vi "Create_Iteration_Data_Files.vi"(7 "Current Iteration":u32, 8 "error in (no error)":errorcluster, 9 "Counter (in)":refnum<class "Counter.lvclass">, 10 "Hamamatsu_C9100-13 (in)":refnum<class "Hamamatsu_C9100-13.lvclass">, 11 "ExperimentVariables in":refnum<class "ExperimentVariables.lvclass">) -> (0 "error out":errorcluster, 1 "Counter out":refnum<class "Counter.lvclass">, 2 "Hamamatsu_C9100-13":refnum<class "Hamamatsu_C9100-13.lvclass">, 3 "ExperimentVariables out":refnum<class "ExperimentVariables.lvclass">)   [LabVIEW 2013]
uses:
  Camera/Hamamatsu_C9100-13/Hamamatsu_C9100-13.lvclass
  Counter/Counter.lvclass
  ExperimentVariables.lvclass
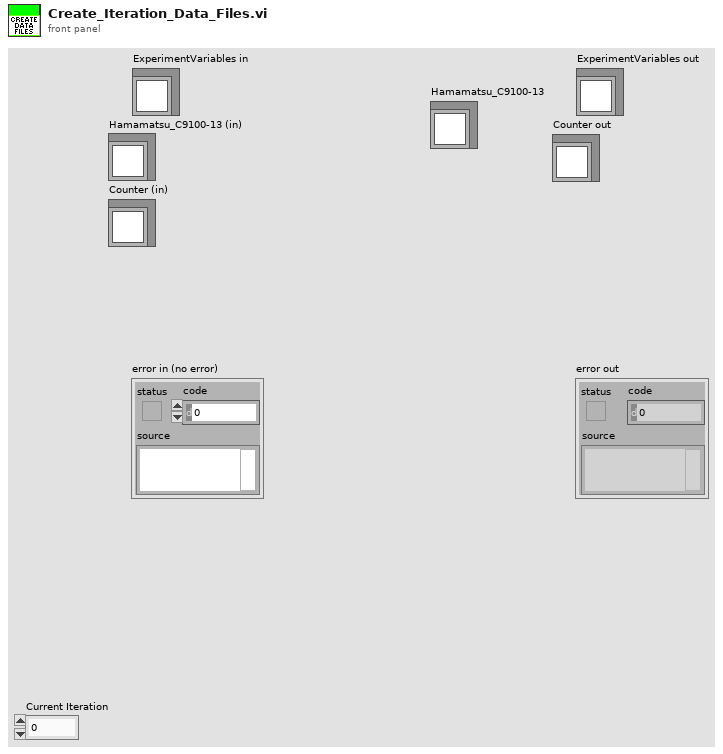
[diagram p1: front panel]
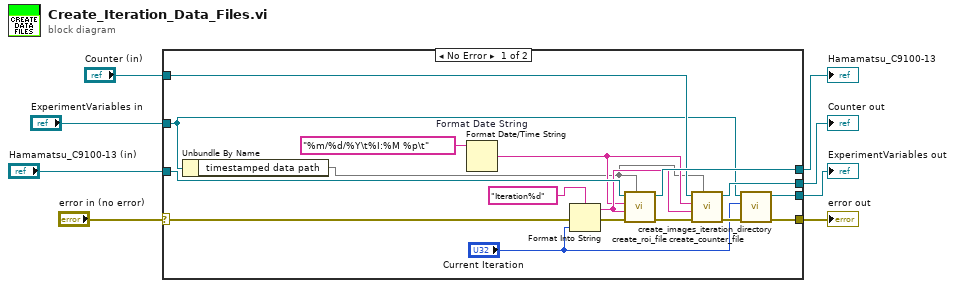
[diagram p0: block diagram]
diagram:
  n1 = case shown="No Error" "error in (no error)" {
    selector: "error in (no error)" -> [w9 w29]
    tunnel: [w14 w29] -> w7
    tunnel: [w12 w28] -> w5
    tunnel: "ExperimentVariables in" -> [w13 w28]
    tunnel: "Hamamatsu_C9100-13 (in)" -> [w23 w27]
    tunnel: [w20 w27] -> w3
    tunnel: "Counter (in)" -> [w19 w26]
    tunnel: [w18 w26] -> w1
    frame No Error {
      n2 = Unbundle By Name(w13) -> ("timestamped data path"=w11)
      n3 = Format Date/Time String "Format Date String"(time format string (%c)="%m/%d/%Y\t%I:%M %p\t") -> (date/time string=w16:string)  [unwired: 2 in]
      n4 = Format Into String(format string="Iteration%d", error in=w9, "Current Iteration") -> (resulting string=w17:string, error out=w22:errorcluster)  [unwired: 1 in]
      n5 = call-dynamic "create_roi_file.vi"("Data Files Path"=w11, "error in (no error)"=w22, "iteration string"=w17, "date/time string"=w16, "Camera in"=w23) -> ("error out"=w21:errorcluster, "Camera out"=w20:refnum<class "Hamamatsu_C9100-13.lvclass">)  [unwired: 5 in]
      n6 = call-dynamic "create_counter_file.vi"("Data Files Path"=w11, "error in (no error)"=w21, "iteration string"=w17, "date/time string"=w16, "Counter in"=w19) -> ("error out"=w15:errorcluster, "Counter out"=w18:refnum<class "Counter.lvclass">)  [unwired: 5 in]
      n7 = call-dynamic "create_images_iteration_directory.vi"("error in (no error)"=w15, "Current Iteration"="Current Iteration", "ExperimentVariables in"=w13) -> ("error out"=w14:errorcluster, "ExperimentVariables out"=w12:refnum<class "ExperimentVariables.lvclass">)  [unwired: 7 in]
    }
    frame Error {
    }
  }
  "error out" <- w7
  "ExperimentVariables out" <- w5
  "Hamamatsu_C9100-13" <- w3
  "Counter out" <- w1
